vi "RGB2Lab.vi"(0 "Image":T1) -> (1 "hang":i32, 4 "lie":i32, 6 "L":dbl[](array[numeric]), 7 "a":dbl[](array[numeric]), 8 "b":dbl[](array[numeric]))   [LabVIEW 2014]
uses:
  <vilib>/vision/Image Controls.llb/IMAQ Image.ctl
  <vilib>/Analysis/Matrix/Datatypes/RealMatrix.ctl
  <vilib>/Analysis/baseanly.llb/Real A x B.vi
  <vilib>/Analysis/NI_AALBase.lvlib
  <vilib>/Analysis/Matrix/NI_Matrix.lvlib
  <vilib>/vision/NI_Vision_Development_Module.lvlib
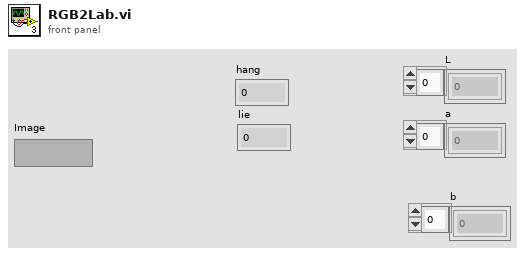
[diagram p1: front panel]
types:
  T1 = typedef "IMAQ Image.ctl" = refnum<image>
  T2 = typedef "Image Type" = u32
  T3 = typedef "NI_Matrix.lvlib/RealMatrix.ctl" = dbl[][]
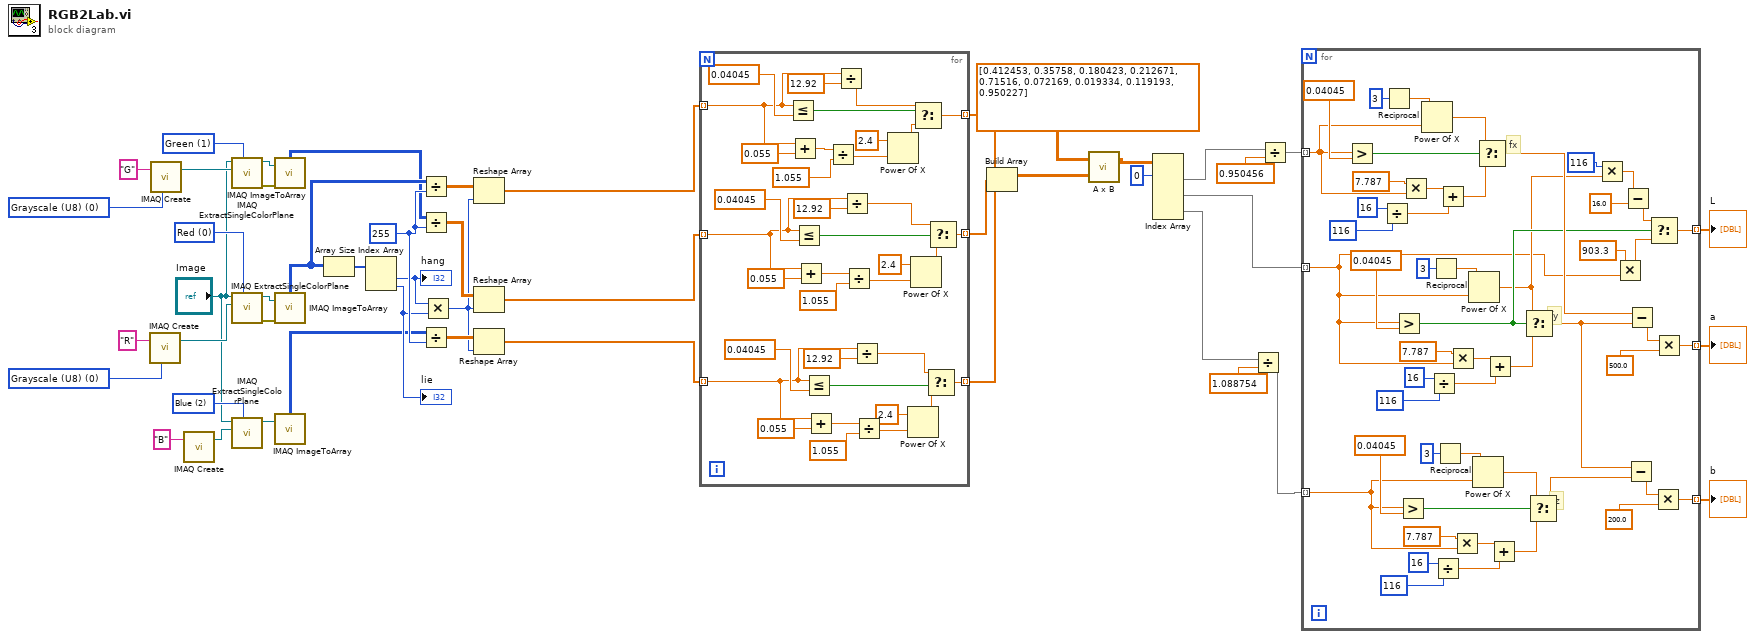
[diagram p0: block diagram]
diagram:
  w9 = T2 0 items=["Grayscale (U8)", "Grayscale (I16)", "Grayscale (SGL)", "Complex (CSG)", "RGB (U32)", "HSL (U32)", "RGB (U64)", "Grayscale (U16)"] ("Image Type")
  w11 = T2 0 items=["Grayscale (U8)", "Grayscale (I16)", "Grayscale (SGL)", "Complex (CSG)", "RGB (U32)", "HSL (U32)", "RGB (U64)", "Grayscale (U16)"] ("Image Type")
  w18 = 1 items=["Red", "Green", "Blue", "Hue", "Saturation", "Luminance", "Value", "Intensity"] ("Color Plane")
  w19 = 0 items=["Red", "Green", "Blue", "Hue", "Saturation", "Luminance", "Value", "Intensity"] ("Color Plane")
  w20 = 2 items=["Red", "Green", "Blue", "Hue", "Saturation", "Luminance", "Value", "Intensity"] ("Color Plane")
  w31 = 255
  n1 = call "IMAQ Create"("Image Name"="R", "Image Type"=w11) -> ("New Image"=w7:T1)  [unwired: 2 in, 2 out]
  n2 = call "IMAQ Create"("Image Name"="G", "Image Type"=w9) -> ("New Image"=w8:T1)  [unwired: 2 in, 2 out]
  n3 = call "IMAQ Create"("Image Name"="B") -> ("New Image"=w1:T1)  [unwired: 3 in, 2 out]
  n4 = call "IMAQ ExtractSingleColorPlane"("Color Plane"=w18, "Image Dst"=w8, "Image Src"="Image") -> ("error out"=w16:errorcluster, "Image Dst Out"=w13:T1)  [unwired: 7 in]
  n5 = call "IMAQ ExtractSingleColorPlane"("Color Plane"=w19, "Image Dst"=w7, "Image Src"="Image") -> ("error out"=w17:errorcluster, "Image Dst Out"=w14:T1)  [unwired: 7 in]
  n6 = call "IMAQ ExtractSingleColorPlane"("Color Plane"=w20, "Image Dst"=w1, "Image Src"="Image") -> ("Image Dst Out"=w15:T1)  [unwired: 7 in, 1 out]
  n7 = call "IMAQ ImageToArray"("error in (no error)"=w16, "Image"=w13) -> ("Image Pixels (U8)"=w4:u8[][])  [unwired: 2 in, 4 out]
  n8 = call "IMAQ ImageToArray"("error in (no error)"=w17, "Image"=w14) -> ("Image Pixels (U8)"=w5:u8[][])  [unwired: 2 in, 4 out]
  n9 = call "IMAQ ImageToArray"("Image"=w15) -> ("Image Pixels (U8)"=w3:u8[][])  [unwired: 3 in, 4 out]
  n10 = Array Size(array=w5) -> (size(s)=w30:i32[])
  n11 = Index Array(array=w30) -> (element #1=w25:i32, element #2=w24:i32)  [unwired: 2 in]
  "hang" <- w25
  "lie" <- w24
  n12 = Divide(x=w5, y=w31) -> (x/y=w28:dbl[][])
  n13 = Divide(x=w4, y=w31) -> (x/y=w29:dbl[][])
  n14 = Divide(x=w3, y=w31) -> (x/y=w27:dbl[][])
  n15 = Multiply(x=w25, y=w24) -> (x*y=w26:i32)
  n16 = Reshape Array(w28, w26) -> (w23:dbl[])
  n17 = Reshape Array(w29, w26) -> (w22:dbl[])
  n18 = Reshape Array(w27, w26) -> (w21:dbl[])
  n19 = for {
    tunnel: w23 -> [w76] mode=indexing
    tunnel: w22 -> [w67] mode=indexing
    tunnel: w21 -> [w58] mode=indexing
    tunnel: [w55] -> w48 mode=indexing
    tunnel: [w50] -> w46 mode=indexing
    tunnel: [w49] -> w47 mode=indexing
    n20 = Less Or Equal?(x=w76, y=0.04045) -> (x <= y?=w83:bool)
    n21 = Add(x=w76, y=0.055) -> (x+y=w80:dbl)
    n22 = Less Or Equal?(x=w67, y=0.04045) -> (x <= y?=w74:bool)
    n23 = Add(x=w67, y=0.055) -> (x+y=w71:dbl)
    n24 = Less Or Equal?(x=w58, y=0.04045) -> (x <= y?=w65:bool)
    n25 = Add(x=w58, y=0.055) -> (x+y=w62:dbl)
    n26 = Divide(x=w80, y=1.055) -> (x/y=w78:dbl)
    n27 = Divide(x=w76, y=12.92) -> (x/y=w57:dbl)
    n28 = Divide(x=w67, y=12.92) -> (x/y=w54:dbl)
    n29 = Divide(x=w71, y=1.055) -> (x/y=w69:dbl)
    n30 = Divide(x=w58, y=12.92) -> (x/y=w52:dbl)
    n31 = Divide(x=w62, y=1.055) -> (x/y=w60:dbl)
    n32 = Power Of X(1:w78, 2:2.4 ("y")) -> (0:w56:dbl)
    n33 = Power Of X(1:w60, 2:2.4 ("y")) -> (0:w51:dbl)
    n34 = Power Of X(1:w69, 2:2.4 ("y")) -> (0:w53:dbl)
    n35 = Select(t=w57, s=w83, f=w56) -> (s? t:f=w55:dbl)
    n36 = Select(t=w52, s=w65, f=w51) -> (s? t:f=w50:dbl)
    n37 = Select(t=w54, s=w74, f=w53) -> (s? t:f=w49:dbl)
  }
  n38 = Build Array(w48, w47, w46) -> (w45:dbl[][])
  n39 = call-poly <vilib>:"A x B.vi"("B"=w45, "A"=T3 [[0.412453, 0.35758, 0.180423], [0.212671, 0.71516, 0.072169], [0.019334, 0.119193, 0.950227]]) -> ("A x B"=w43:T3)  [unwired: 1 out]
  n40 = Index Array(array=w43, index (row) #1=0 ("索引 (行)")) -> (element #1=w41:dbl[], element #2=w36:dbl[], element #3=w38:dbl[])  [unwired: 5 in]
  n41 = Divide(x=w38, y=1.088754) -> (x/y=w35:dbl[])
  n42 = Divide(x=w41, y=0.950456) -> (x/y=w37:dbl[])
  n43 = for {
    tunnel: w37 -> [w132] mode=indexing
    tunnel: w36 -> [w87] mode=indexing
    tunnel: w35 -> [w106] mode=indexing
    tunnel: [w102] -> w33 mode=indexing
    tunnel: [w97] -> w32 mode=indexing
    tunnel: [w85] -> w34 mode=indexing
    # "fz"
    # "fy"
    # "fx"
    n44 = Greater?(x=w132, y=0.04045) -> (0:w96:bool)
    n45 = Divide(x=16, y=116) -> (x/y=w128:dbl)
    n46 = Reciprocal(x=3) -> (1/x=w134:dbl)
    n47 = Greater?(x=w87, y=0.04045) -> (0:w89:bool)
    n48 = Greater?(x=w106, y=0.04045) -> (0:w117:bool)
    n49 = Multiply(x=7.787, y=w132) -> (x*y=w131:dbl)
    n50 = Power Of X(1:w132, 2:w134) -> (0:w94:dbl)
    n51 = Divide(x=16, y=116) -> (x/y=w119:dbl)
    n52 = Reciprocal(x=3) -> (1/x=w124:dbl)
    n53 = Divide(x=16, y=116) -> (x/y=w109:dbl)
    n54 = Reciprocal(x=3) -> (1/x=w114:dbl)
    n55 = Add(x=w131, y=w128) -> (x+y=w127:dbl)
    n56 = Multiply(x=7.787, y=w87) -> (x*y=w122:dbl)
    n57 = Multiply(x=7.787, y=w106) -> (x*y=w112:dbl)
    n58 = Power Of X(1:w87, 2:w124) -> (0:w88:dbl)
    n59 = Power Of X(1:w106, 2:w114) -> (0:w107:dbl)
    n60 = Select(t=w94, s=w96, f=w127) -> (s? t:f=w105:dbl)
    n61 = Add(x=w122, y=w119) -> (x+y=w118:dbl)
    n62 = Add(x=w112, y=w109) -> (x+y=w108:dbl)
    n63 = Select(t=w88, s=w89, f=w118) -> (s? t:f=w99:dbl)
    n64 = Select(t=w107, s=w117, f=w108) -> (s? t:f=w98:dbl)
    n65 = Multiply(x=116, y=w88) -> (x*y=w92:dbl)
    n66 = Multiply(x=903.3, y=w87) -> (x*y=w86:dbl)
    n67 = Subtract(x=w92, y=16.0) -> (x-y=w93:dbl)
    n68 = Subtract(x=w99, y=w98) -> (x-y=w100:dbl)
    n69 = Subtract(x=w105, y=w99) -> (x-y=w103:dbl)
    n70 = Select(t=w93, s=w89, f=w86) -> (s? t:f=w85:dbl)
    n71 = Multiply(x=w100, y=200.0) -> (x*y=w97:dbl)
    n72 = Multiply(x=w103, y=500.0) -> (x*y=w102:dbl)
  }
  "L" <- w34
  "a" <- w33
  "b" <- w32
